vi "setLocalAndHold_00.vi"(1 "error in (no error)":errorcluster) -> (0 "error out":errorcluster)   [LabVIEW 2011]
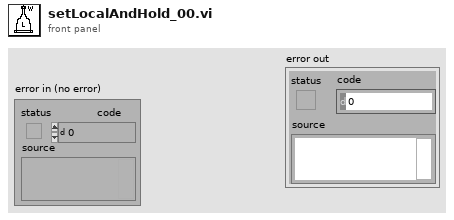
[diagram p1: front panel]
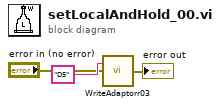
[diagram p0: block diagram]
diagram:
  n1 = call "WriteAdaptorr03.vi"("error in (no error)"="error in (no error)", "string to write"="D5") -> ("error out"=→"error out":errorcluster)
